vi "Write Temp Units.vi"(8 "error in (no error)":errorcluster, 10 "Temp Units":T1, 11 "Temp Chamber in":refnum<class "Temp Chamber.lvclass">) -> (0 "error out":errorcluster, 3 "Temp Chamber out":refnum<class "Temp Chamber.lvclass">)   [LabVIEW 2018, in "Temp Chamber.lvlib" / "Temp Chamber.lvclass"]
uses:
  Temp Chamber.lvclass
  Custom Controls/Temp Units.ctl
  Temp Chamber.lvclass/Temp Chamber.ctl
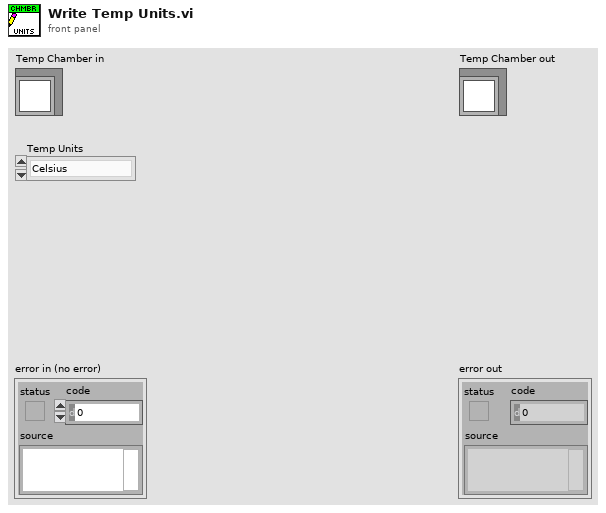
[diagram p1: front panel]
types:
  T1 = typedef "Temp Chamber.lvlib/Temp Chamber.lvclass/Temp Units.ctl" = enum16{"Celsius", "Fahrenheit", "Kelvin", "Rankine"}
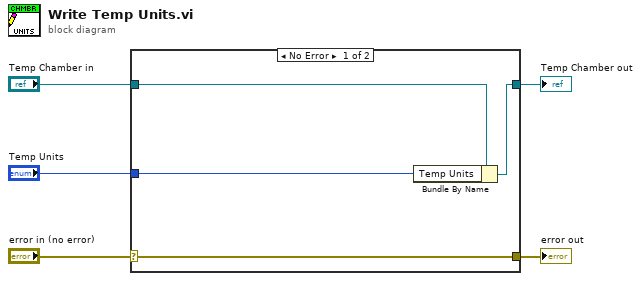
[diagram p0: block diagram]
diagram:
  n1 = case shown="No Error" "error in (no error)" {
    selector: "error in (no error)" -> [w9 w10]
    tunnel: [w9 w10] -> w4
    tunnel: [w7 w11] -> w2
    tunnel: "Temp Chamber in" -> [w8 w11]
    tunnel: "Temp Units" -> [w6 _]
    frame No Error {
      n2 = Bundle By Name(cluster=w8, "Temp Units"=w6) -> (w7:refnum<class "Temp Chamber.lvclass">)
    }
    frame Error {
    }
  }
  "error out" <- w4
  "Temp Chamber out" <- w2
